vi "new crossing available.vi"(7 "don't wait":bool, 8 "error in (no error)":errorcluster, 11 "timeout in ms (-1)":i32=20) -> (0 "error out":errorcluster, 1 "new odd crossing":bool, 2 "new crossing":bool, 3 "crossing stats":T1 {"recent crossing" format="%.4f"})   [LabVIEW 2017]
uses:
  typedefs/crossing stats.ctl
  popup panels/control panel globals.vi
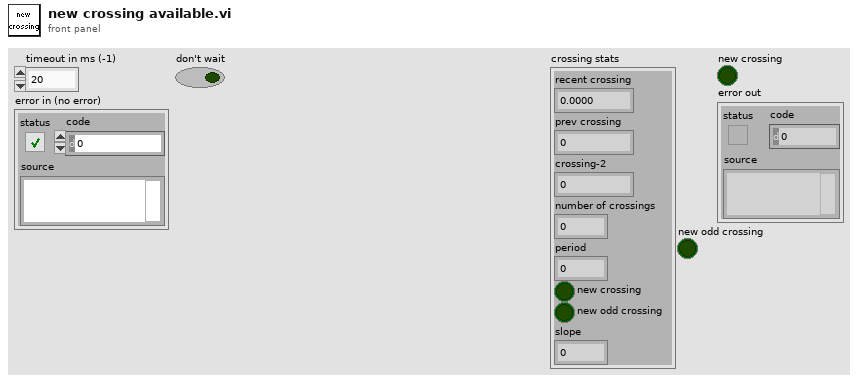
[diagram p1: front panel]
types:
  T1 = typedef "crossing stats.ctl" = cluster{"recent crossing":dbl, "prev crossing":dbl, "crossing-2":dbl, "number of crossings":i32, "period":dbl, "new crossing":bool, "new odd crossing":bool, "slope":dbl}
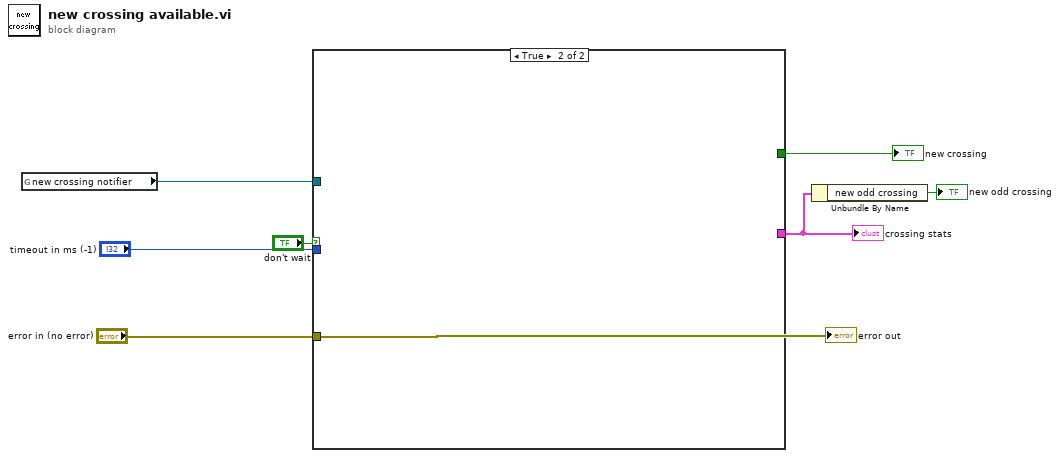
[diagram p0: block diagram]
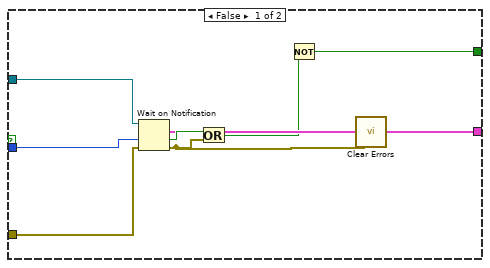
[diagram p2: hidden frame]
diagram:
  n1 = global read "control panel globals.vi" "new crossing notifier"() -> (w4:refnum<notifier>)
  n2 = case shown="True" "don't wait" {
    tunnel: "timeout in ms (-1)" -> [w15 _]
    tunnel: [w12 _] -> w2
    tunnel: [w10 _] -> w6
    tunnel: "error in (no error)" -> [w9 _]
    tunnel: w4 -> [w8 _]
    frame False {
      n3 = Wait on Notification(notifier=w8, timeout in ms (-1)=w15, error in (no error)=w9) -> (notification=w12:T1, timed out?=w14:bool, error out=w13:errorcluster)  [unwired: 1 in, 1 out]
      n4 = Or(x=w14, y=w13) -> (x .or. y?=w11:bool)
      n5 = Not(x=w11) -> (.not. x?=w10:bool)
      n6 = call <vilib>:"Clear Errors.vi"("error in (no error)"=w13) -> ()  [unwired: 5 in, 2 out]
    }
    frame True {
    }
  }
  "new crossing" <- w6
  "crossing stats" <- w2
  n7 = Unbundle By Name(w2) -> ("new odd crossing"=→"new odd crossing":bool)
  "error out" <- "error in (no error)"
